vi "Read Wfm Data.vi"(8 "error in":errorcluster, 11 "Async State Vars in":T1) -> (0 "error out":errorcluster, 3 "Async State Vars out":T1, 4 "Wfm timed out?":bool)   [LabVIEW 2017, in "Waveform-Processing-Custom-Device Engine.lvlib"]
uses:
  Waveform-Processing-Custom-Device Engine.lvlib
  Types/AsyncStateVariables.ctl
  <vilib>/NI VeriStand/Custom Device Waveform API/Single Waveform Read (DBL)/Single Waveform Read (DBL).lvclass
  C:/Program Files (x86)/National Instruments/LabVIEW 2017/vi.lib/NI Veristand/Custom Device Waveform API/Waveform Session.lvclass
  <vilib>/NI VeriStand/Custom Device Waveform API/Single Waveform Write (DBL)/Single Waveform Write (DBL).lvclass
  <vilib>/NI Veristand/Custom Device API/Waveform Data Reference.ctl
  Types/New Async FIFOs.ctl
  <vilib>/NI/NIVS Inline Async API/_Data Access Engine/Data Access Engine/Types/Write.DVR.ctl
  <vilib>/NI/NIVS Inline Async API/_Data Access Engine/Access Type Classes/Write/Write.lvclass
  <userlib>/Circular Buffer/Controls/Circular Buffer Operations.ctl
  <vilib>/NI Veristand/Custom Device Waveform API/Waveform Session.lvclass/Waveform Session.ctl
  <vilib>/NI VeriStand/Custom Device Waveform API/Single Waveform Read (DBL)/Single Waveform Read (DBL).lvclass/Single Waveform Read (DBL).ctl
  <vilib>/NI VeriStand/Custom Device Waveform API/Internal Comm Classes/WPL Comm/WPL Comm (1D DBL)/WPL Comm (1D DBL).lvclass/WPL Comm (1D DBL).ctl
  <vilib>/NI Veristand/Custom Device Waveform API/Single Waveform Read (DBL)/NI VeriStand - Read Single Waveform (DBL).vi
  <vilib>/NI Veristand/Custom Device Waveform API/Internal Comm Classes/WPL Comm/WPL Comm (1D DBL)/Comm_read 1d dbl.vi
  <vilib>/NI Veristand/Custom Device Waveform API/Check Opened.vi
  <vilib>/NI Veristand/Custom Device Waveform API/Internal Comm Classes/WPL Comm/Convert Q Error to Shutdown Error.vi
  <vilib>/Utility/error.llb/Error Cluster From Error Code.vi
  <userlib>/Circular Buffer/Instance VIs/Circular Buffer(2D DBL).vi
  <vilib>/NI Veristand/Custom Device Waveform API/NI_VS Custom Device Waveform API.lvlib
  <userlib>/Circular Buffer/Circular Buffer.lvlib
  <vilib>/NI Veristand/Custom Device API/Custom Device API.lvlib
  <vilib>/NI/NIVS Inline Async API/_Data Access Engine/Data Access Engine/Data Access Engine.lvclass
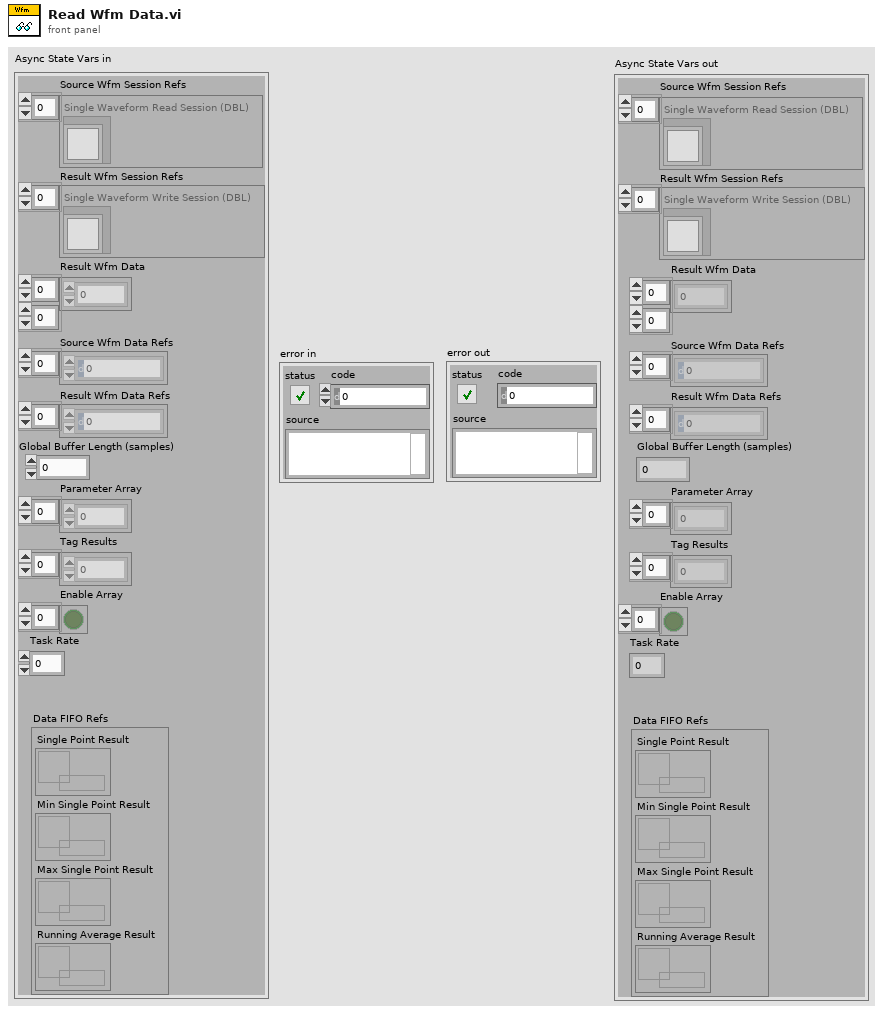
[diagram p1: front panel]
types:
  T1 = typedef "Waveform-Processing-Custom-Device Engine.lvlib/AsyncStateVariables.ctl" = cluster{"Source Wfm Session Refs":refnum<class "Single Waveform Read (DBL).lvclass">[], "Result Wfm Session Refs":refnum<class "Single Waveform Write (DBL).lvclass">[], "Result Wfm Data":dbl[][], "Source Wfm Data Refs":T2[], "Result Wfm Data Refs":T2[], "Global Buffer Length (samples)":dbl, "Parameter Array":dbl[], "Tag Results":dbl[], "Enable Array":bool[], "Task Rate":dbl, "Data FIFO Refs":T3}
  T2 = typedef "Custom Device API.lvlib/Waveform Data Reference.ctl" = i32
  T3 = typedef "Waveform-Processing-Custom-Device Engine.lvlib/New Async FIFOs.ctl" = cluster{"Single Point Result":T4, "Running Average Result":T4, "Min Single Point Result":T4, "Max Single Point Result ":T4}
  T4 = typedef "Data Access Engine.lvlib/Data Access Engine.lvclass/Write.DVR.ctl" = refnum<data-value>
  T5 = typedef "Circular Buffer.lvlib/Circular Buffer Operations.ctl" = enum16{"Initialize", "Get Backlog", "Write", "Read (continuous)", "Read (most recent)"}
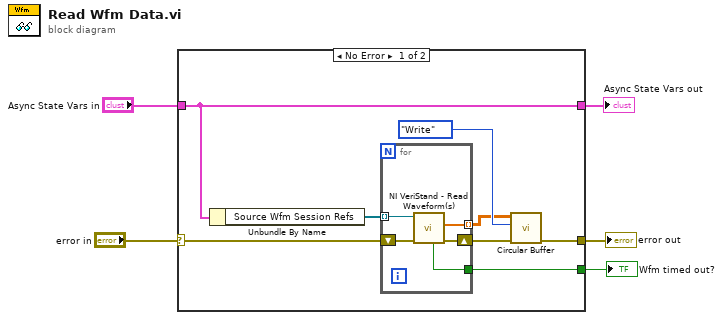
[diagram p0: block diagram]
diagram:
  n1 = case shown="No Error" "error in" {
    selector: "error in" -> [w9 w19]
    tunnel: [w10 w19] -> w5
    tunnel: "Async State Vars in" -> [w8 w20]
    tunnel: [w8 w20] -> w2
    tunnel: [w7 _] -> w1
    frame No Error {
      n2 = Unbundle By Name(w8) -> ("Source Wfm Session Refs"=w13:refnum<class "Single Waveform Read (DBL).lvclass">[])
      n3 = for {
        tunnel: [w16] -> w6 mode=indexing
        tunnel: [w15] -> w7
        tunnel: w13 -> [w14] mode=indexing
        shift-right: [w17] -> w12
        shift-left: w9 -> [w18]
        n4 = call-poly <vilib>:"NI VeriStand - Read Waveform(s).vi"("error in (no error)"=w18, "Single Waveform Read Session (DBL) in"=w14) -> ("error out"=w17:errorcluster, "Data"=w16:dbl[], "timed out?"=w15:bool)  [unwired: 5 in, 2 out]
      }
      n5 = call-poly <userlib>:"Circular Buffer.vi"("error in (no error)"=w12, "Operation"=Circular_Buffer_Operations."Write", "Data In"=w6) -> ("error out"=w10:errorcluster)  [unwired: 5 in, 3 out]
    }
    frame Error {
    }
  }
  "error out" <- w5
  "Wfm timed out?" <- w1
  "Async State Vars out" <- w2
